vi "I2C_WriteWordData.vi"(4 "Word":u16 format="%.0x", 5 "Bus":i32=1, 6 "Device register":u8 format="%.0x", 7 "Address":u8 format="%.0x", 8 "error in":errorcluster) -> (0 "error out":errorcluster)   [LabVIEW 2014]
doc: "Read a single word from the specified I2C device and register"
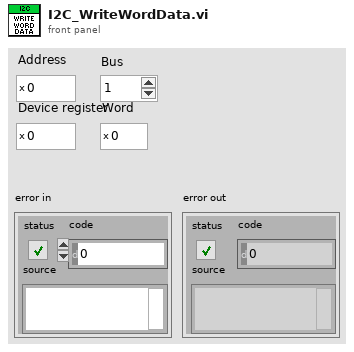
[diagram p1: front panel]
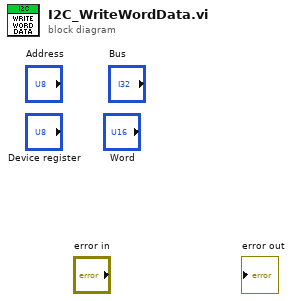
[diagram p0: block diagram]
diagram:
